vi "ControlSystemLaser.vi"() -> ()   [LabVIEW 2012]
uses:
  SingleControls/TypeDef_LoopStages.ctl
  GlobalVariables_DIALMain.vi
  <vilib>/Utility/miscctls.llb/LVRectTypeDef.ctl
  <vilib>/Utility/miscctls.llb/LVPointTypeDef.ctl
  SingleControls/TypeDef_LaserTypes.ctl
  SingleControls/TypeDef_LaserControl.ctl
  SingleControls/TypeDef_LaserIndicator.ctl
panel:
  in  "Scan Sequence":dbl[](array[numeric])=[0.0, 3.0, 2.0, 0.0, 3.0, 1.0, 0.0, 3.0, 2.0, 0.0, 3.0, 4.0]
  out "Laser Indicator":T1[](array[typedef])
  in  "Laser Control":T2[](array[typedef])=[{"I Gain"=0.0, "D Gain"=0.0, "P Gain"=0.0, "Locking Tol."=0.0, "Wavelength "=0.0, "Temperature "=0.0, "Current "=0.0, "Detector Types"=enum."WV Online"}, {"I Gain"=0.0, "D Gain"=0.0, "P Gain"=0.0, "Locking Tol."=0.0, "Wavelength "=0.0, "Temperature "=0.0, "Current "=0.0, "Detector Types"=enum."WV Offline"}, {"I Gain"=0.0, "D Gain"=0.0, "P Gain"=0.0, "Locking Tol."=0.0, "Wavelength "=0.0, "Temperature "=0.0, "Current "=0.0, "Detector Types"=enum."HSRL"}, {"I Gain"=0.0, "D Gain"=0.0, "P Gain"=0.0, "Locking Tol."=0.0, "Wavelength "=0.0, "Temperature "=0.0, "Current "=0.0, "Detector Types"=enum."O2 Online"}, {"I Gain"=0.0, "D Gain"=0.0, "P Gain"=0.0, "Locking Tol."=0.0, "Wavelength "=0.0, "Temperature "=0.0, "Current "=0.0, "Detector Types"=enum."O2 Offline"}]
  out "Commands Executed":i32
  in  "Reset Plot Bounds":bool
  out "Local Loop Stage":T4=enum."Exit"
  out "Total Errors":i32
  out "Permission Level":T5(ring)
  out "Local Queue Response":string="Exit Idle Loop"
  in  "Replot":bool
  in  "User Comment":bool
  in  "Update Permissions":bool
  in  "Software Testing":bool
  in  "Commanded Abort":bool
  out "Waiting Commands":i32
  out "Local Queue Element":string="Exit"
  in  "Local Abort":bool=TRUE
  # "Place Hidden Variables Here"
  # "Place Global Buttons Here"
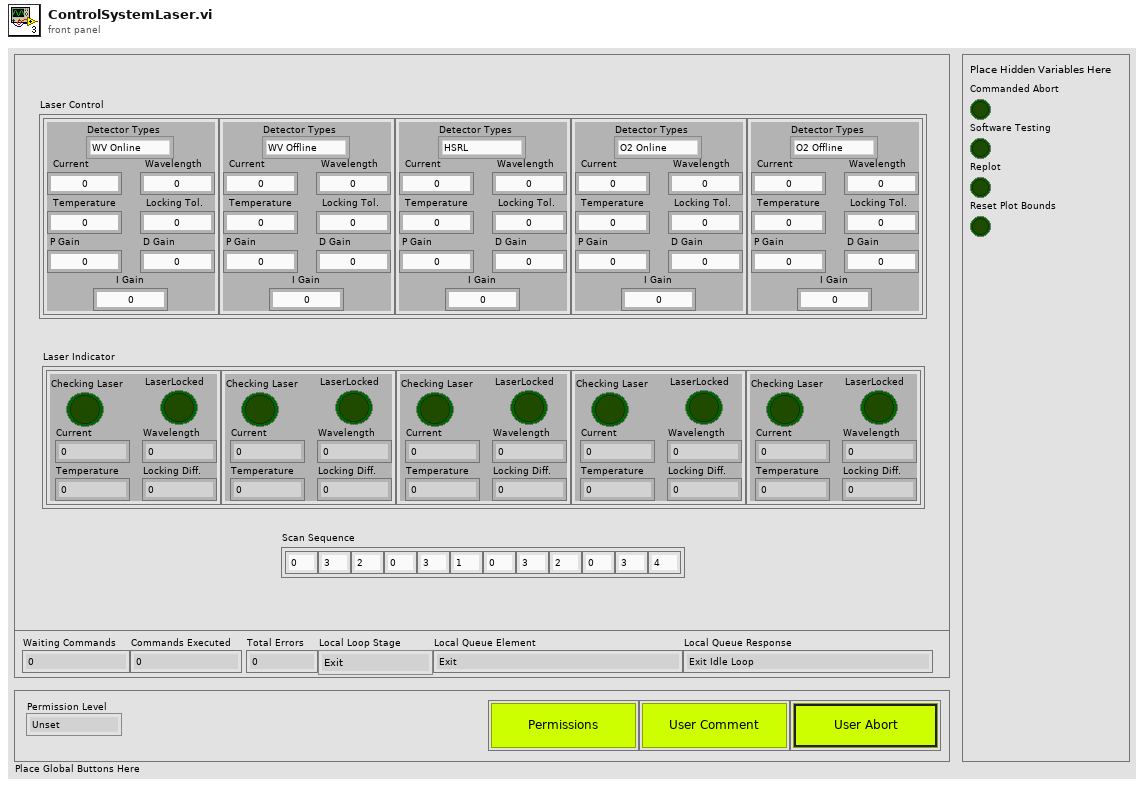
[diagram p1: front panel]
types:
  T1 = typedef "TypeDef_LaserIndicator.ctl" = cluster{"Locking Diff.":dbl, "Wavelength":dbl, "Temperature":dbl, "Current ":dbl, "LaserLocked":bool, "Checking Laser":bool}
  T2 = typedef "TypeDef_LaserControl.ctl" = cluster{"I Gain":dbl, "D Gain":dbl, "P Gain":dbl, "Locking Tol.":dbl, "Wavelength ":dbl, "Temperature ":dbl, "Current ":dbl, "Detector Types":T3}
  T3 = typedef "TypeDef_LaserTypes.ctl" = enum16{"WV Online", "WV Offline", "HSRL", "O2 Online", "O2 Offline"}
  T4 = typedef "TypeDef_LoopStages.ctl" = enum16{"Configure", "Initialize", "Idle", "Error Handler", "Commanded Exit", "Exit"}
  T5 = enum16{"Unset", "Operator", "Administrator", "Full"}
  T6 = typedef "LVPointTypeDef.ctl" = cluster{"Horizontal":i16, "Vertical":i16}
  T7 = typedef "LVRectTypeDef.ctl" = cluster{"Left":i16, "Top":i16, "Right":i16, "Bottom":i16}
  T8 = enum16{"Always On", "Always Off", "Off While Running"}
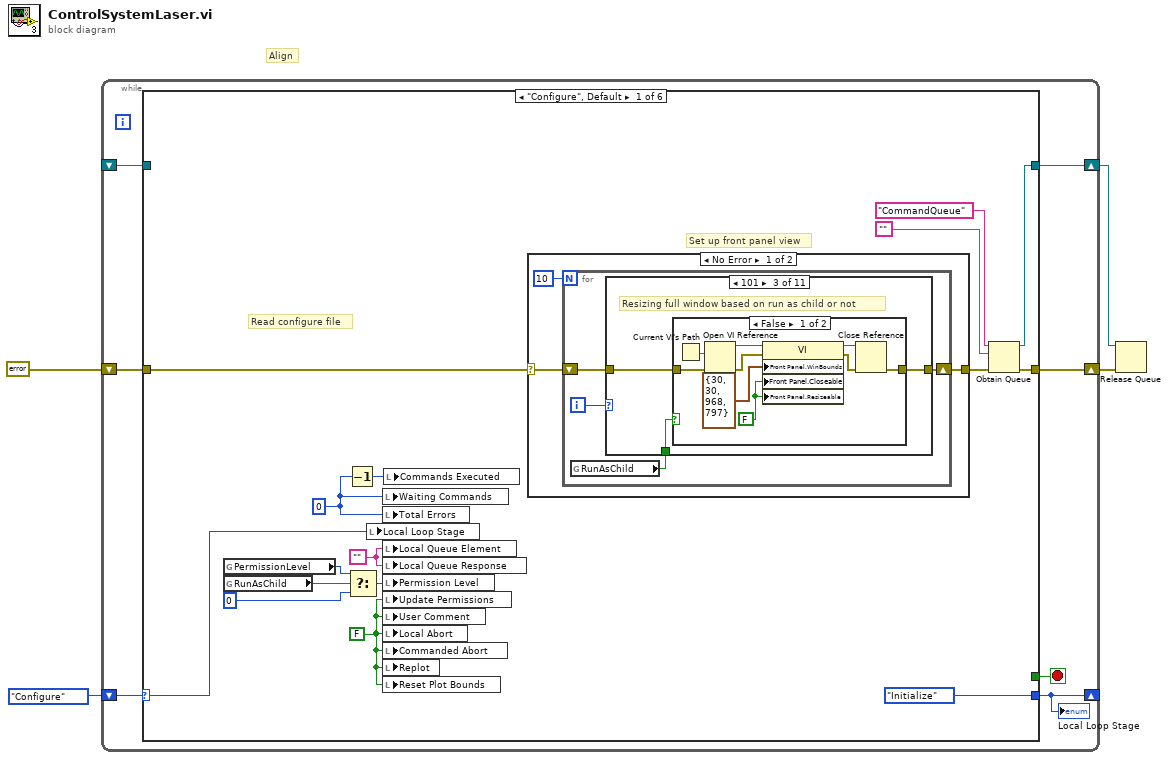
[diagram p0: block diagram]
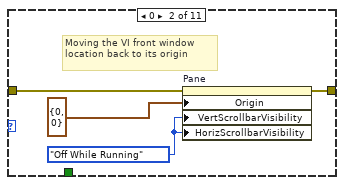
[diagram p3: hidden frame]
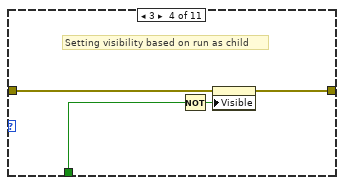
[diagram p5: hidden frame]
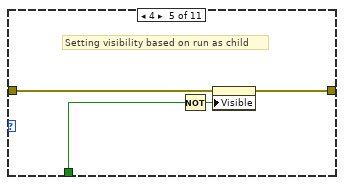
[diagram p6: hidden frame]
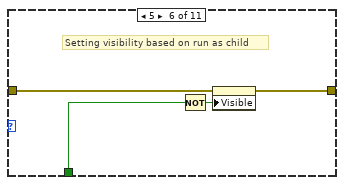
[diagram p7: hidden frame]
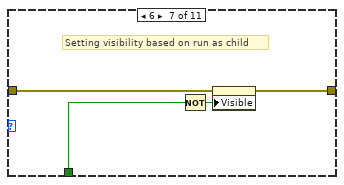
[diagram p8: hidden frame]
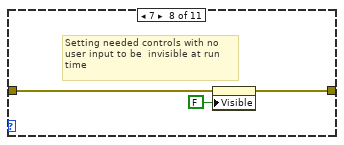
[diagram p9: hidden frame]
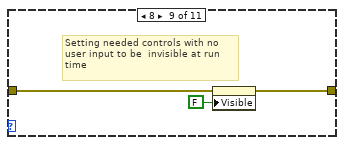
[diagram p10: hidden frame]
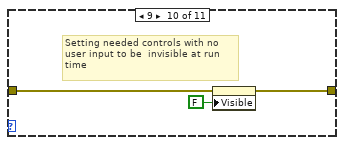
[diagram p11: hidden frame]
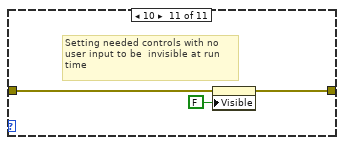
[diagram p12: hidden frame]
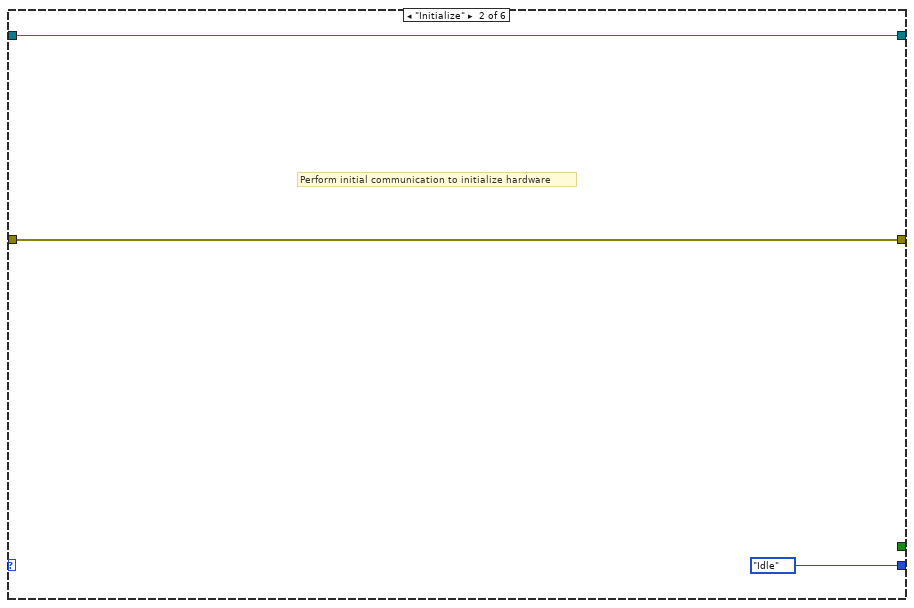
[diagram p14: hidden frame]
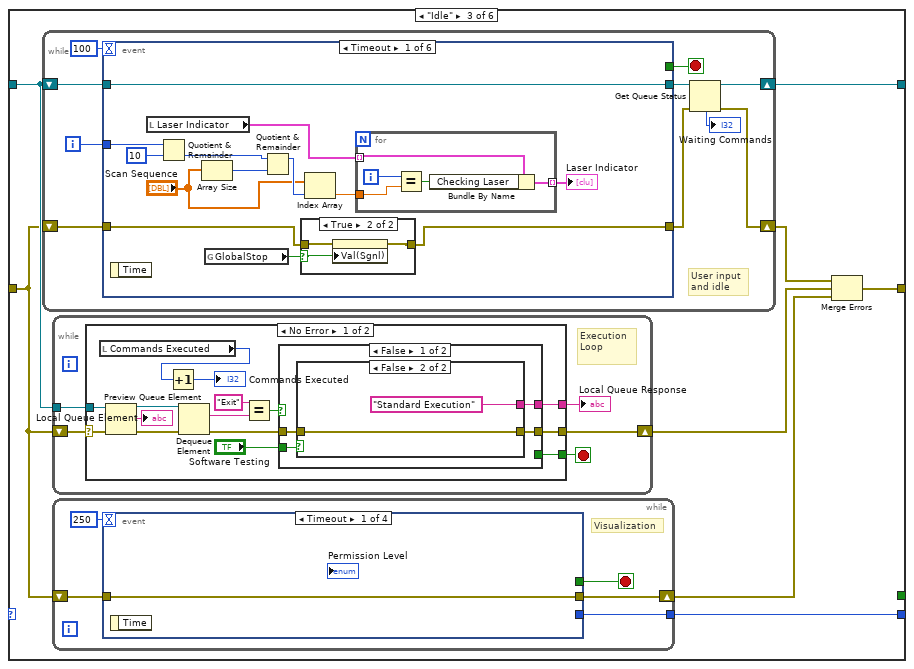
[diagram p15: hidden frame]
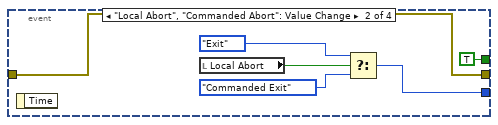
[diagram p16: hidden frame]
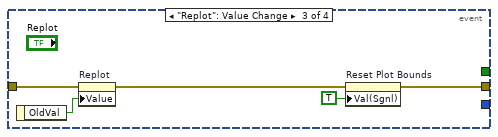
[diagram p17: hidden frame]
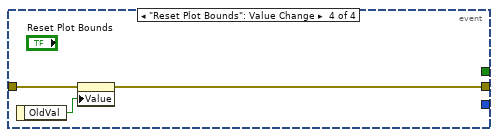
[diagram p18: hidden frame]
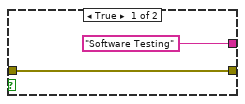
[diagram p19: hidden frame]
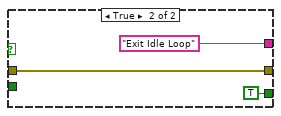
[diagram p20: hidden frame]
diagram:
  # "Align"
  n1 = while {
    shift-right: [w10] -> _
    shift-left: TypeDef_LoopStages."Configure" ("Enum") -> [w11]
    shift-right: [w8] -> w1
    shift-left: errorcluster {"status"=FALSE, "code"=0, "source"=""} ("error out") -> [w6]
    shift-right: [w7] -> w2
    shift-left: _ -> [w5]
    stop <- w9 stop-if-true
    n2 = case shown="\"Configure\", Default" w11 {
      selector: w11 -> [w21 _ _ _ _ _]
      tunnel: [TypeDef_LoopStages."Initialize" ("Enum") TypeDef_LoopStages."Idle" ("Enum") w85 TypeDef_LoopStages."Exit" ("Enum") TypeDef_LoopStages."Exit" ("Enum") TypeDef_LoopStages."Exit" ("Enum")] -> w10
      tunnel: [_ _ _ _ TRUE TRUE] -> w9
      tunnel: [w26 w83 w89 w208 w212 w215] -> w8
      tunnel: [w25 w82 w88 w209 w213 w217] -> w7
      tunnel: w6 -> [w14 w83 w87 w208 w212 w216]
      tunnel: w5 -> [_ w82 w92 w209 w213 w217]
      frame "Configure", Default {
        w13 = 0 ("Waiting Commands")
        w19 = FALSE ("Local Abort")
        w20 = ""
        # "Read configure file"
        # "Set up front panel view"
        n3 = global read "GlobalVariables_DIALMain.vi" "PermissionLevel"() -> (w17:i32)
        n4 = global read "GlobalVariables_DIALMain.vi" "RunAsChild"() -> (w18:bool)
        n5 = Decrement(x=w13) -> (x-1=w12:i32)
        n6 = Select(t=w17, s=w18, f=0) -> (s? t:f=w15:i32)
        n7 = local write "Local Loop Stage"(w21) -> ()
        n8 = local write "Waiting Commands"(w13) -> ()
        n9 = local write "Total Errors"(w13) -> ()
        n10 = local write "Local Queue Element"(w20) -> ()
        n11 = local write "Local Queue Response"(w20) -> ()
        n12 = local write "Permission Level"(w15) -> ()
        n13 = local write "Update Permissions"(w19) -> ()
        n14 = local write "User Comment"(w19) -> ()
        n15 = local write "Local Abort"(w19) -> ()
        n16 = local write "Commanded Abort"(w19) -> ()
        n17 = local write "Replot"(w19) -> ()
        n18 = local write "Reset Plot Bounds"(w19) -> ()
        n19 = local write "Commands Executed"(w12) -> ()
        n20 = case shown="No Error" w14 {
          selector: w14 -> [w30 w81]
          tunnel: [w29 w81] -> w22
          frame No Error {
            n21 = for {
              N: 10 -> [_]
              shift-right: [w32] -> w29
              shift-left: w30 -> [w33]
              i -> [w34]
              n22 = global read "GlobalVariables_DIALMain.vi" "RunAsChild"() -> (w31:bool)
              n23 = case shown="101" w34 {
                tunnel: w33 -> [w35 w38 w42 w54 w60 w63 w66 w70 w73 w76 w79]
                tunnel: [w35 w37 w41 w55 w59 w64 w67 w71 w74 w77 w80] -> w32
                tunnel: w31 -> [_ _ w40 w56 w57 w61 w68 _ _ _ _]
                frame -1, Default {
                }
                frame 0 {
                  w36 = T8."Off While Running" ("Vertical Scrollbar Visibility")
                  # "Moving the VI front window location back to its origin"
                  n24 = property on="Pane" class="Pane"(error in=w38, "Origin"=T6 {"Horizontal"=0, "Vertical"=0}, "VertScrollbarVisibility"=w36, "HorizScrollbarVisibility"=w36) -> (error out=w37:errorcluster)  [unwired: 1 in, 1 out]
                }
                frame 101 {
                  # "Resizing full window based on run as child or not"
                  n25 = case shown="False" w40 {
                    tunnel: w42 -> [w50 w52]
                    tunnel: [w45 w52] -> w41
                    frame False {
                      w43 = FALSE
                      n26 = Current VI's Path() -> (path=w51:path)
                      n27 = Open VI Reference(vi path=w51, error in (no error)=w50) -> (vi reference=w49:refnum<vi>, error out=w48:errorcluster)  [unwired: 4 in]
                      n28 = property class="VI"(reference=w49, error in=w48, "Front Panel.WinBounds"=T7 {"Left"=30, "Top"=30, "Right"=968, "Bottom"=797} ("Front Panel Window:Panel Bounds"), "Front Panel.Closeable"=w43, "Front Panel.Resizeable"=w43) -> (reference out=w47:refnum<vi>, error out=w46:errorcluster)
                      n29 = Close Reference(reference=w47, error in (no error)=w46) -> (error out=w45:errorcluster)
                    }
                    frame True {
                    }
                  }
                }
                frame 3 {
                  # "Setting visibility based on run as child"
                  n30 = Not(x=w56) -> (.not. x?=w53:bool)
                  n31 = property on="Permission Level" class="Enum (strict)"(error in=w54, "Visible"=w53) -> (error out=w55:errorcluster)  [unwired: 1 in, 1 out]
                }
                frame 4 {
                  # "Setting visibility based on run as child"
                  n32 = Not(x=w57) -> (.not. x?=w58:bool)
                  n33 = property on="Update Permissions" class="Bool (strict)"(error in=w60, "Visible"=w58) -> (error out=w59:errorcluster)  [unwired: 1 in, 1 out]
                }
                frame 5 {
                  # "Setting visibility based on run as child"
                  n34 = Not(x=w61) -> (.not. x?=w62:bool)
                  n35 = property on="User Comment" class="Bool (strict)"(error in=w63, "Visible"=w62) -> (error out=w64:errorcluster)  [unwired: 1 in, 1 out]
                }
                frame 6 {
                  # "Setting visibility based on run as child"
                  n36 = Not(x=w68) -> (.not. x?=w65:bool)
                  n37 = property on="Local Abort" class="Bool (strict)"(error in=w66, "Visible"=w65) -> (error out=w67:errorcluster)  [unwired: 1 in, 1 out]
                }
                frame 7 {
                  # "Setting needed controls with no user input to be  invisible at run time"
                  n38 = property on="Commanded Abort" class="Bool (strict)"(error in=w70, "Visible"=FALSE) -> (error out=w71:errorcluster)  [unwired: 1 in, 1 out]
                }
                frame 8 {
                  # "Setting needed controls with no user input to be  invisible at run time"
                  n39 = property on="Software Testing" class="Bool (strict)"(error in=w73, "Visible"=FALSE) -> (error out=w74:errorcluster)  [unwired: 1 in, 1 out]
                }
                frame 9 {
                  # "Setting needed controls with no user input to be  invisible at run time"
                  n40 = property on="Replot" class="Bool (strict)"(error in=w76, "Visible"=FALSE) -> (error out=w77:errorcluster)  [unwired: 1 in, 1 out]
                }
                frame 10 {
                  # "Setting needed controls with no user input to be  invisible at run time"
                  n41 = property on="Reset Plot Bounds" class="Bool (strict)"(error in=w79, "Visible"=FALSE) -> (error out=w80:errorcluster)  [unwired: 1 in, 1 out]
                }
              }
            }
          }
          frame Error {
          }
        }
        n42 = Obtain Queue(name (unnamed)="CommandQueue", element data type="", error in (no error)=w22) -> (queue out=w25:refnum<queue>, error out=w26:errorcluster)  [unwired: 2 in, 1 out]
      }
      frame "Initialize" {
        # "Perform initial communication to initialize hardware"
      }
      frame "Idle" {
        n43 = while {
          shift-right: [w152] -> w88
          shift-left: w92 -> [w156]
          shift-right: [w150] -> w91
          shift-left: w87 -> [w155]
          i -> [w148]
          stop <- w154 stop-if-true
          # "User input\nand idle"
          n44 = event shown="[0] Timeout" {
            selector: _ -> [_ _ _ _ _ _]
            dyn-events: _ -> [_ _ _ _ _ _]
            timeout: 100 -> [_ _ _ _ _ _]
            tunnel: w156 -> [w170 w185 w191 w193 w202 w207]
            tunnel: [w170 w184 w187 w194 w198 w203] -> w153
            tunnel: w155 -> [w162 w181 w189 w196 w200 w205]
            tunnel: [w161 w180 w188 w195 w199 w204] -> w151
            tunnel: [_ _ TRUE ("LocalAbort") TRUE ("LocalAbort") _ _] -> w154
            tunnel: w148 -> [w159 _ _ _ _ _]
            event Timeout {
              n45 = event-data() -> ()  [unwired: 1 in, 1 out]
              n46 = local read "Laser Indicator"() -> (w166:T1[])
              n47 = Quotient & Remainder(x=w159, y=10) -> (floor(x/y)=w158:i32)  [unwired: 1 out]
              n48 = Array Size(array="Scan Sequence") -> (size(s)=w169:i32)
              n49 = global read "GlobalVariables_DIALMain.vi" "GlobalStop"() -> (w163:bool)
              n50 = Quotient & Remainder(x=w158, y=w169) -> (x-y*floor(x/y)=w168:i32)  [unwired: 1 out]
              n51 = case shown="True" w163 {
                selector: w163 -> [_ w172]
                tunnel: w162 -> [w171 w173]
                tunnel: [w171 w174] -> w161
                frame False {
                }
                frame True {
                  n52 = property on="Commanded Abort" class="Bool (strict)"(error in=w173, "Val(Sgnl)"=w172) -> (error out=w174:errorcluster)  [unwired: 1 in, 1 out]
                }
              }
              n53 = Index Array(array="Scan Sequence", index=w168) -> (element=w167:dbl)
              n54 = for {
                tunnel: w166 -> [w179] mode=indexing
                tunnel: w167 -> [w177]
                tunnel: [w175] -> w164 mode=indexing
                i -> [w178]
                n55 = Equal?(x=w178, y=w177) -> (x = y?=w176:bool)
                n56 = Bundle By Name(cluster=w179, "Checking Laser"=w176) -> (w175:T1)
              }
              "Laser Indicator" <- w164
            }
            event "Laser Control": Value Change {
              n57 = event-data() -> ("OldVal"=w183:T2[], "NewVal"=w182:T2[])  [unwired: 1 in]
              n58 = call "Idle_MakeCommandLaser.vi"("Error In"=w181, "Laser Control New"=w182, "Laser Control Old"=w183, "Queue In"=w185) -> ("Error Out"=w180:errorcluster, "Queue Out"=w184:refnum<queue>)  [unwired: 5 in, 1 out]
            }
            event "Local Abort": Value Change {
              n59 = event-data() -> ()  [unwired: 1 in, 1 out]
              n60 = Enqueue Element At Opposite End(queue=w191, element="Exit", error in (no error)=w189) -> (queue out=w187:refnum<queue>, error out=w188:errorcluster)  [unwired: 1 in, 1 out]
            }
            event "Commanded Abort": Value Change {
              n61 = event-data() -> ()  [unwired: 1 in, 1 out]
              n62 = Enqueue Element At Opposite End(queue=w193, element="Exit", error in (no error)=w196) -> (queue out=w194:refnum<queue>, error out=w195:errorcluster)  [unwired: 1 in, 1 out]
            }
            event "Update Permissions": Value Change {
              n63 = event-data() -> ()  [unwired: 1 in, 1 out]
              n64 = Enqueue Element(queue=w202, element="System_OpenPermissionsVI", error in (no error)=w200) -> (queue out=w198:refnum<queue>, error out=w199:errorcluster)  [unwired: 1 in, 1 out]
            }
            event "User Comment": Value Change {
              n65 = event-data() -> ()  [unwired: 1 in, 1 out]
              n66 = Enqueue Element(queue=w207, element="System_OpenUserCommentVI", error in (no error)=w205) -> (queue out=w203:refnum<queue>, error out=w204:errorcluster)  [unwired: 1 in, 1 out]
            }
          }
          n67 = Get Queue Status(queue=w153, error in (no error)=w151) -> (queue out=w152:refnum<queue>, error out=w150:errorcluster, # elements in queue=→"Waiting Commands":i32)  [unwired: 1 in, 5 out]
        }
        n68 = while {
          tunnel: w92 -> [w115]
          shift-right: [w116] -> w90
          shift-left: w87 -> [w114]
          stop <- w117 stop-if-true
          # "Execution Loop"
          n69 = case shown="No Error" w114 {
            selector: w114 -> [w122 w147]
            tunnel: [w130 _] -> w117
            tunnel: [w125 w147] -> w116
            tunnel: w115 -> [w124 _]
            tunnel: [w120 "Error Loop Entered"] -> w113
            frame No Error {
              n70 = local read "Commands Executed"() -> (w119:i32)
              n71 = Preview Queue Element(queue=w124, error in (no error)=w122) -> (queue out=w123:refnum<queue>, element=→"Local Queue Element":string, error out=w132:errorcluster)  [unwired: 1 in, 1 out]
              n72 = Increment(x=w119) -> (x+1=→"Commands Executed":i32)
              n73 = Dequeue Element(queue=w123, error in (no error)=w132) -> (element=w126:string, error out=w127:errorcluster)  [unwired: 1 in, 2 out]
              n74 = Equal?(x="Exit", y=w126) -> (x = y?=w129:bool)
              n75 = case shown="False" w129 {
                tunnel: w127 -> [w135 w142]
                tunnel: [w134 w142] -> w125
                tunnel: "Software Testing" -> [w136 _]
                tunnel: [_ TRUE] -> w130
                tunnel: [w133 "Exit Idle Loop"] -> w120
                frame False {
                  n76 = case shown="False" w136 {
                    tunnel: w135 -> [w138 w140]
                    tunnel: [w138 w140] -> w134
                    tunnel: ["Software Testing" "Standard Execution"] -> w133
                    frame True {
                    }
                    frame False {
                    }
                  }
                }
                frame True {
                }
              }
            }
            frame Error {
              n77 = local read "Total Errors"() -> (w144:i32)
              n78 = Increment(x=w144) -> (x+1=→"Total Errors":i32)
            }
          }
          "Local Queue Response" <- w113
        }
        n79 = while {
          shift-right: [w95] -> w86
          shift-left: w87 -> [w96]
          tunnel: [w93] -> w85
          stop <- w94 stop-if-true
          # "Visualization"
          n80 = event shown="[0] Timeout" {
            selector: _ -> [_ _ _ _]
            dyn-events: _ -> [_ _ _ _]
            timeout: 250 -> [_ _ _ _]
            tunnel: w96 -> [w98 w103 w107 w112]
            tunnel: [w98 w103 w109 w111] -> w95
            tunnel: [_ TRUE ("LocalAbort") _ _] -> w94
            tunnel: [_ w99 _ _] -> w93
            event Timeout {
              n81 = event-data() -> ()  [unwired: 1 in, 1 out]
            }
            event "Local Abort", "Commanded Abort": Value Change {
              n82 = event-data() -> ()  [unwired: 1 in, 1 out]
              n83 = local read "Local Abort"() -> (w102:bool)
              n84 = Select(t=TypeDef_LoopStages."Exit" ("Enum"), s=w102, f=TypeDef_LoopStages."Commanded Exit" ("Enum")) -> (s? t:f=w99:T4)
            }
            event "Replot": Value Change {
              n85 = event-data() -> ("OldVal"=w105:bool)  [unwired: 1 in]
              n86 = property on="Replot" class="Bool (strict)"(error in=w107, "Value"=w105) -> (error out=w106:errorcluster)  [unwired: 1 in, 1 out]
              n87 = property on="Reset Plot Bounds" class="Bool (strict)"(error in=w106, "Val(Sgnl)"=TRUE ("Value (Signaling)")) -> (error out=w109:errorcluster)  [unwired: 1 in, 1 out]
            }
            event "Reset Plot Bounds": Value Change {
              n88 = event-data() -> ("OldVal"=w110:bool)  [unwired: 1 in]
              n89 = property on="Reset Plot Bounds" class="Bool (strict)"(error in=w112, "Value"=w110) -> (error out=w111:errorcluster)  [unwired: 1 in, 1 out]
            }
          }
        }
        n90 = Merge Errors(w91, w90, w86) -> (w89:errorcluster)
      }
      frame "Error Handler" {
      }
      frame "Commanded Exit" {
      }
      frame "Exit" {
        n91 = case shown="No Error" w216 {
          selector: w216 -> [w222 w252]
          tunnel: [w221 w252] -> w215
          frame No Error {
            n92 = for {
              N: 8 -> [_]
              shift-right: [w224] -> w221
              shift-left: w222 -> [w225]
              i -> [w226]
              n93 = case shown="-1, Default" w226 {
                tunnel: w225 -> [w227 w229 w232 w235 w238 w241 w244 w247 w250]
                tunnel: [w227 w230 w233 w236 w239 w242 w245 w248 w251] -> w224
                tunnel: TRUE ("Visible") -> [_ w228 w231 w234 w237 w240 w243 w246 w249]
                frame -1, Default {
                }
                frame 0 {
                  n94 = property on="Permission Level" class="Enum (strict)"(error in=w229, "Visible"=w228) -> (error out=w230:errorcluster)  [unwired: 1 in, 1 out]
                }
                frame 1 {
                  n95 = property on="Update Permissions" class="Bool (strict)"(error in=w232, "Visible"=w231) -> (error out=w233:errorcluster)  [unwired: 1 in, 1 out]
                }
                frame 2 {
                  n96 = property on="User Comment" class="Bool (strict)"(error in=w235, "Visible"=w234) -> (error out=w236:errorcluster)  [unwired: 1 in, 1 out]
                }
                frame 3 {
                  n97 = property on="Local Abort" class="Bool (strict)"(error in=w238, "Visible"=w237) -> (error out=w239:errorcluster)  [unwired: 1 in, 1 out]
                }
                frame 4 {
                  n98 = property on="Commanded Abort" class="Bool (strict)"(error in=w241, "Visible"=w240) -> (error out=w242:errorcluster)  [unwired: 1 in, 1 out]
                }
                frame 5 {
                  n99 = property on="Software Testing" class="Bool (strict)"(error in=w244, "Visible"=w243) -> (error out=w245:errorcluster)  [unwired: 1 in, 1 out]
                }
                frame 6 {
                  n100 = property on="Replot" class="Bool (strict)"(error in=w247, "Visible"=w246) -> (error out=w248:errorcluster)  [unwired: 1 in, 1 out]
                }
                frame 7 {
                  n101 = property on="Reset Plot Bounds" class="Bool (strict)"(error in=w250, "Visible"=w249) -> (error out=w251:errorcluster)  [unwired: 1 in, 1 out]
                }
              }
            }
          }
          frame Error {
          }
        }
      }
    }
    "Local Loop Stage" <- w10
  }
  n102 = Release Queue(queue=w2, error in (no error)=w1) -> ()  [unwired: 1 in, 3 out]
